vi "Read NombrePruebas 2.vi"(8 "error in (no error)":errorcluster, 11 "Dosimetro in":refnum<class "Dosimetro.lvclass">) -> (0 "error out":errorcluster, 2 "NombrePruebas":string[](array[string]), 3 "Dosimetro out":refnum<class "Dosimetro.lvclass">)   [LabVIEW 2019, in "Dosimetro.lvclass"]
uses:
  Dosimetro.lvclass
  Dosimetro.lvclass/Dosimetro.ctl
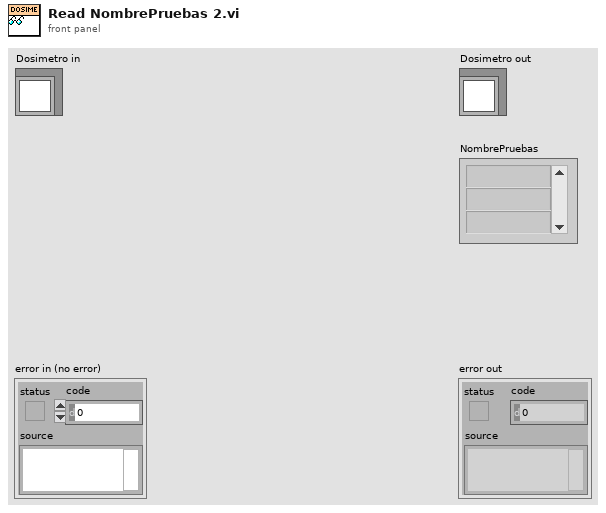
[diagram p1: front panel]
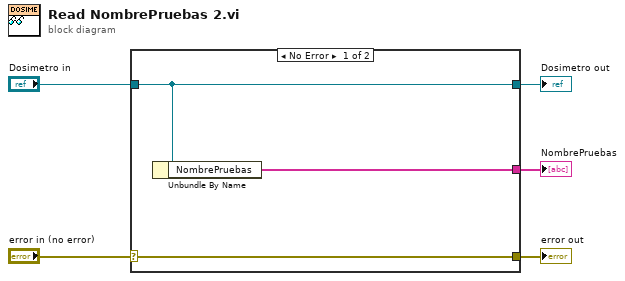
[diagram p0: block diagram]
diagram:
  n1 = case shown="No Error" "error in (no error)" {
    selector: "error in (no error)" -> [w8 w9]
    tunnel: [w8 w9] -> w4
    tunnel: [w7 w10] -> w2
    tunnel: "Dosimetro in" -> [w7 w10]
    tunnel: [w6 _] -> w1
    frame No Error {
      n2 = Unbundle By Name(w7) -> ("NombrePruebas"=w6:string[])
    }
    frame Error {
    }
  }
  "error out" <- w4
  "Dosimetro out" <- w2
  "NombrePruebas" <- w1
